vi "gyro safety data toggle display.vi"(0 "Select Gyro":bool, 1 "Select Safeties":bool, 2 "Select Robot Data":bool, 3 "Select Quick Settings":bool, 4 "Select LED Control":bool) -> (11 "Button States":cluster{bool, bool, bool, bool, bool}, 13 "Change of State":bool, 14 "Gyro Visibility":bool, 15 "Safety Visibility":bool, 16 "Robot Data Visibility":bool, 17 "Quick Settings Visibility":bool, 18 "LED Control Visibility":bool)   [LabVIEW 2014]
panel:
  out "LED Control Button State":bool
  out "Gyro Button State":bool
  out "Safety Button State":bool
  out "Robot Data Button State":bool
  out "Quick Settings Button State":bool
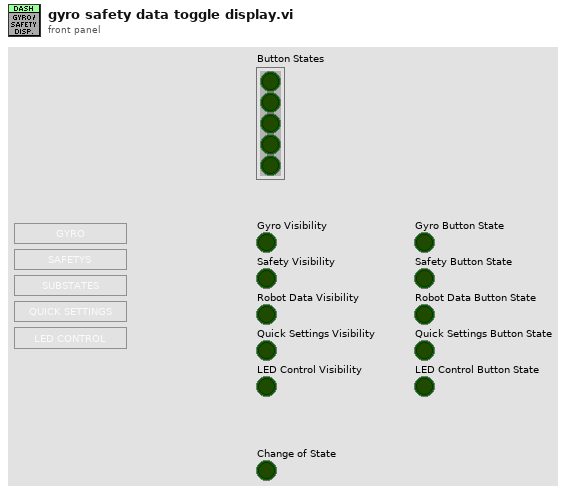
[diagram p1: front panel]
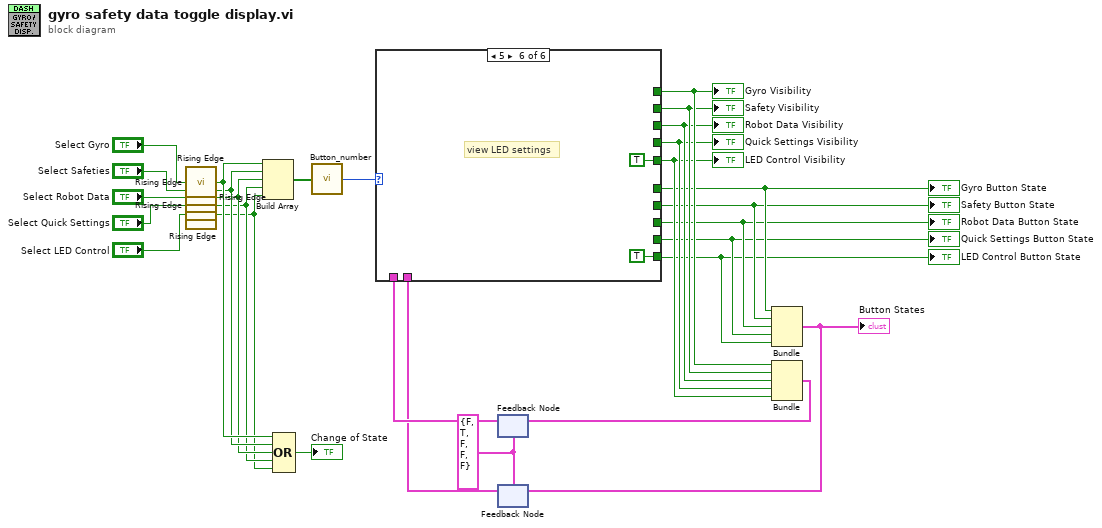
[diagram p0: block diagram]
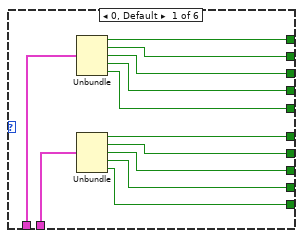
[diagram p2: hidden frame]
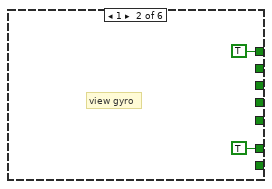
[diagram p3: hidden frame]
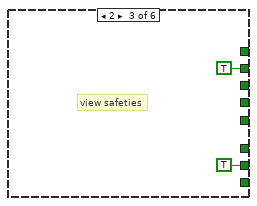
[diagram p4: hidden frame]
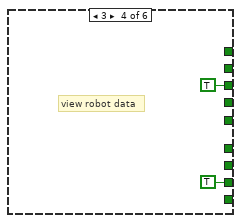
[diagram p5: hidden frame]
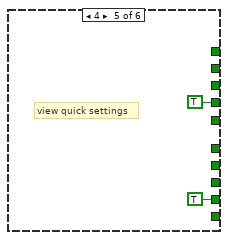
[diagram p6: hidden frame]
diagram:
  w7 = cluster{bool, bool, bool, bool, bool} {FALSE, TRUE, FALSE, FALSE, FALSE}
  n1 = call "Rising Edge.vi"("Input"="Select Gyro") -> ("Rising Edge"=w17:bool)
  n2 = call "Rising Edge.vi"("Input"="Select Safeties") -> ("Rising Edge"=w16:bool)
  n3 = call "Rising Edge.vi"("Input"="Select Robot Data") -> ("Rising Edge"=w15:bool)
  n4 = call "Rising Edge.vi"("Input"="Select Quick Settings") -> ("Rising Edge"=w14:bool)
  n5 = call "Rising Edge.vi"("Input"="Select LED Control") -> ("Rising Edge"=w8:bool)
  n6 = Build Array(w17, w16, w15, w14, w8) -> (w13:bool[])
  n7 = Compound Arithmetic op=OR(w17, w16, w15, w14, w8) -> (→"Change of State":bool)
  n8 = call "Button_number.vi"("Button Array"=w13) -> ("Button Pressed"=w23:i32)
  n9 = feedback #1(w7) -> (w18:cluster{bool, bool, bool, bool, bool})
  n10 = feedback #2(w7) -> (w10:cluster{bool, bool, bool, bool, bool})
  n11 = case shown="5" w23 {
    tunnel: [w39 TRUE _ _ _ _] -> w22
    tunnel: [w38 _ TRUE _ _ _] -> w21
    tunnel: [w37 _ _ TRUE _ _] -> w20
    tunnel: [w36 _ _ _ TRUE _] -> w19
    tunnel: [w34 TRUE _ _ _ _] -> w5
    tunnel: [w33 _ TRUE _ _ _] -> w4
    tunnel: [w32 _ _ TRUE _ _] -> w3
    tunnel: [w31 _ _ _ TRUE _] -> w2
    tunnel: w18 -> [w40 _ _ _ _ _]
    tunnel: w10 -> [w35 _ _ _ _ _]
    tunnel: [w30 _ _ _ _ TRUE] -> w6
    tunnel: [w29 _ _ _ _ TRUE] -> w1
    frame 0, Default {
      n12 = Unbundle(w40) -> (w39:bool, w38:bool, w37:bool, w36:bool, w30:bool)
      n13 = Unbundle(w35) -> (w34:bool, w33:bool, w32:bool, w31:bool, w29:bool)
    }
    frame 1 {
      # "view gyro"
    }
    frame 2 {
      # "view safeties"
    }
    frame 3 {
      # "view robot data"
    }
    frame 4 {
      # "view quick settings"
    }
    frame 5 {
      # "view LED settings"
    }
  }
  "Gyro Visibility" <- w22
  "Safety Visibility" <- w21
  "Robot Data Visibility" <- w20
  "Quick Settings Visibility" <- w19
  "Gyro Button State" <- w5
  "Safety Button State" <- w4
  "Robot Data Button State" <- w3
  "Quick Settings Button State" <- w2
  "LED Control Visibility" <- w6
  "LED Control Button State" <- w1
  n14 = Bundle(w5, w4, w3, w2, w1) -> (w11:cluster{bool, bool, bool, bool, bool})  [unwired: 1 in]
  "Button States" <- w11
  n15 = feedback-in #2(w11) -> ()
  n16 = Bundle(w22, w21, w20, w19, w6) -> (w12:cluster{bool, bool, bool, bool, bool})  [unwired: 1 in]
  n17 = feedback-in #1(w12) -> ()
